vi "Send_Message.vi"(8 "error in (no error)":errorcluster, 10 "message":T1={"message data"=variant, "message type"=enum."Stop"}, 11 "connection ID":refnum<k5>) -> (0 "error out (no error)":errorcluster, 1 "TX":bool, 3 "connection ID 2":refnum<k5>)   [LabVIEW 2013]
uses:
  Messages.ctl
  messageTypes.ctl
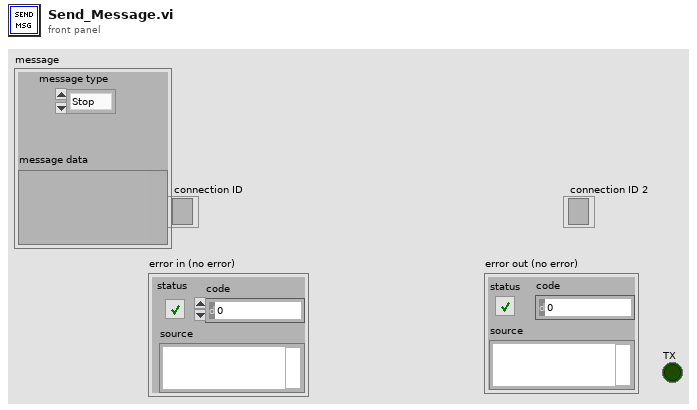
[diagram p1: front panel]
types:
  T1 = typedef "Messages.ctl" = cluster{"message data":variant, "message type":T2}
  T2 = typedef "messageTypes.ctl" = enum16{"Speeds", "Stop", "PolarCoordinates", "Gains", "Setpoints"}
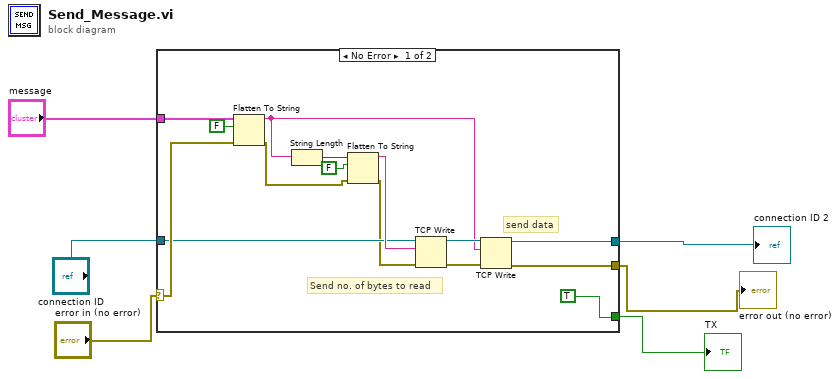
[diagram p0: block diagram]
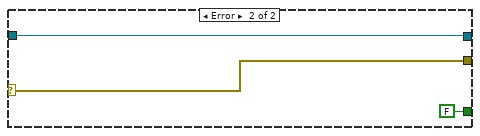
[diagram p2: hidden frame]
diagram:
  n1 = case shown="No Error" "error in (no error)" {
    selector: "error in (no error)" -> [w20 w24]
    tunnel: [w10 w24] -> w4
    tunnel: "message" -> [w21 _]
    tunnel: "connection ID" -> [w16 w23]
    tunnel: [w9 w23] -> w5
    tunnel: [TRUE FALSE] -> w6
    frame No Error {
      # "send data"
      # "Send no. of bytes to read"
      n2 = Flatten To String(anything=w21, prepend array or string size? (T)=FALSE, error in (no error)=w20) -> (data string=w14:string, error out=w13:errorcluster)  [unwired: 1 in, 1 out]
      n3 = String Length(string=w14) -> (length=w18:i32)
      n4 = Flatten To String(anything=w18, prepend array or string size? (T)=FALSE, error in (no error)=w13) -> (data string=w17:string, error out=w12:errorcluster)  [unwired: 1 in, 1 out]
      n5 = TCP Write(connection ID=w16, data in=w17, error in (no error)=w12) -> (connection ID out=w15:refnum<k5>, error out=w11:errorcluster)  [unwired: 1 in, 1 out]
      n6 = TCP Write(connection ID=w15, data in=w14, error in (no error)=w11) -> (connection ID out=w9:refnum<k5>, error out=w10:errorcluster)  [unwired: 1 in, 1 out]
    }
    frame Error {
    }
  }
  "error out (no error)" <- w4
  "connection ID 2" <- w5
  "TX" <- w6
